vi "msg.vi"(9 "F button name (\"Cancel\")":string, 10 "T button name (\"OK\")":string, 11 "message":string) -> (3 "T button?":bool)   [LabVIEW 2013, in "DeviceInterface.lvclass"]
uses:
  DeviceInterface.lvclass
panel:
  in  "false":bool
  in  "true":bool
  out "message 2":string
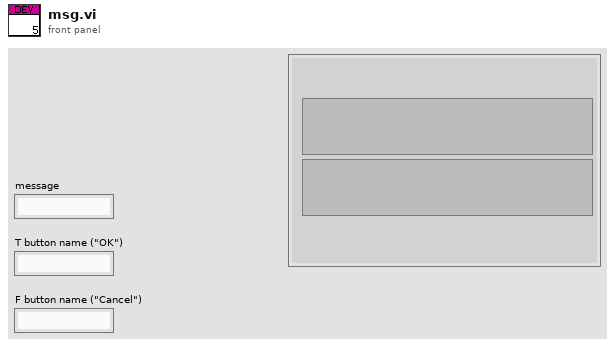
[diagram p1: front panel]
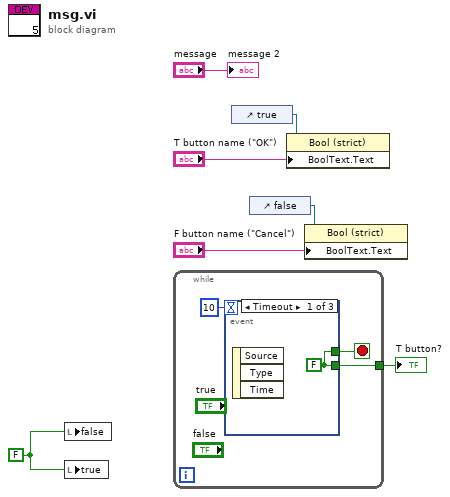
[diagram p0: block diagram]
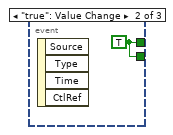
[diagram p2: hidden frame]
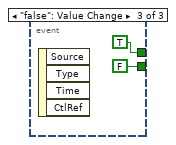
[diagram p3: hidden frame]
diagram:
  w1 = FALSE
  n1 = local write "false"(w1) -> ()
  n2 = local write "true"(w1) -> ()
  n3 = while {
    tunnel: [w8] -> w2
    stop <- w9 stop-if-true
    n4 = event shown="[0] Timeout" {
      selector: _ -> [_ _ _]
      dyn-events: _ -> [_ _ _]
      timeout: 10 -> [_ _ _]
      tunnel: [w11 w12 TRUE] -> w9
      tunnel: [w11 w12 FALSE] -> w8
      event Timeout {
        w11 = FALSE
        n5 = event-data() -> ()  [unwired: 1 in, 3 out]
      }
      event "true": Value Change {
        w12 = TRUE
        n6 = event-data() -> ()  [unwired: 1 in, 4 out]
      }
      event "false": Value Change {
        n7 = event-data() -> ()  [unwired: 1 in, 4 out]
      }
    }
  }
  "T button?" <- w2
  n8 = control-ref of="true"() -> (w5:refnum<vi>)
  n9 = control-ref of="false"() -> (w6:refnum<vi>)
  n10 = property class="Bool (strict)"(reference=w5, "BoolText.Text"="T button name (\"OK\")") -> ()  [unwired: 1 in, 2 out]
  n11 = property class="Bool (strict)"(reference=w6, "BoolText.Text"="F button name (\"Cancel\")") -> ()  [unwired: 1 in, 2 out]
  "message 2" <- "message"
